vi "Set Double Message.vi"(7 "Format":string, 8 "error in (no error)":errorcluster, 9 "Value":dbl, 10 "Name":string, 11 "Message Double in":refnum<class "Message Double.lvclass">) -> (0 "error out":errorcluster, 3 "Message Double out":refnum<class "Message Double.lvclass">)   [LabVIEW 2016, in "Stream Mediator.lvlib" / "Message Double.lvclass"]
doc: "--\nCopyright © 2017 Composed SystemsI All rights reserved.\n\nAuthor: Jon McBee <jon.mcbee@composed.io>\n\nThis library is provided \"AS IS\" ,WITHOUT WARRANTIES OR\nCONDITIONS OF ANY KIND, either express or implied.\n\nComposed Systems -- composed.io\n\nStream 0.0.1.1\nJon McBee - Composed Systems\nCopyright (c) 2017, Composed Systems"
uses:
  <userlib>/Composed Systems/Stream/Mediator/Classes/Message Double/Message Double.lvclass
  C:/Program Files (x86)/National Instruments/LabVIEW 2016/user.lib/Composed Systems/Stream/Mediator/Classes/Message Interface/Message Interface.lvclass
  <userlib>/Composed Systems/Stream/Mediator/Classes/Message Double/Message Double.lvclass/Message Double.ctl
  <userlib>/Composed Systems/Stream/Mediator/Classes/Message Interface/Message Interface.lvclass
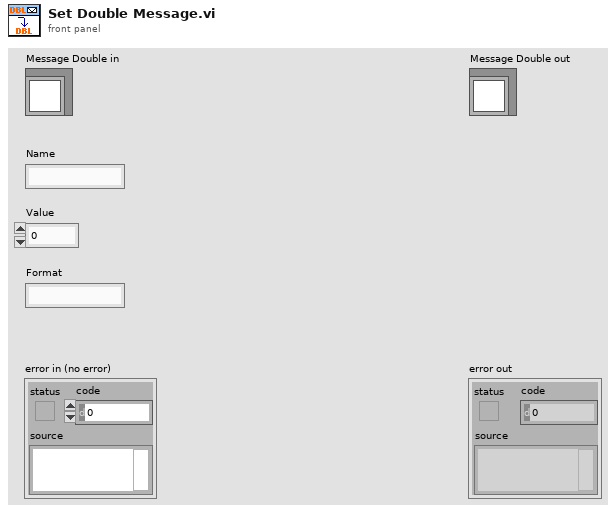
[diagram p1: front panel]
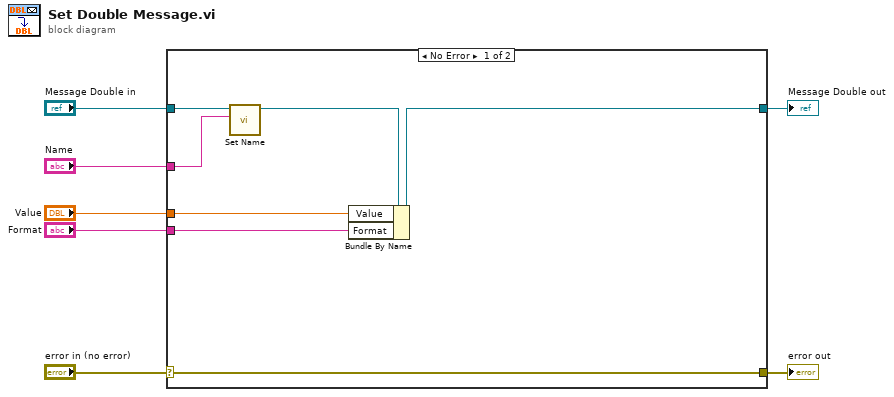
[diagram p0: block diagram]
diagram:
  n1 = case shown="No Error" "error in (no error)" {
    selector: "error in (no error)" -> [w14 w16]
    tunnel: [w14 w16] -> w6
    tunnel: [w10 w15] -> w4
    tunnel: "Message Double in" -> [w13 w15]
    tunnel: "Name" -> [w12 _]
    tunnel: "Value" -> [w9 _]
    tunnel: "Format" -> [w8 _]
    frame No Error {
      n2 = call <userlib>:"Set Name.vi"("Name"=w12, "Message Interface in"=w13) -> ("Message Interface out"=w11:refnum<class "Message Double.lvclass">)  [unwired: 8 in, 1 out]
      n3 = Bundle By Name(cluster=w11, "Value"=w9, "Format"=w8) -> (w10:refnum<class "Message Double.lvclass">)
    }
    frame Error {
    }
  }
  "error out" <- w6
  "Message Double out" <- w4
